vi "CAN read.vi"(8 "error in":errorcluster, 11 "CANopen in":refnum<class "CANopen.lvclass">) -> (0 "error out":errorcluster, 1 "Data":u8[](array[numeric]), 2 "COB-ID":u32, 3 "CANopen out":refnum<class "CANopen.lvclass">, 5 "Time Stamp":timestamp)   [LabVIEW 2024, in "canopen.lvlib" / "CANopen.lvclass"]
doc: "Returns the oldest COB present in the reception queue."
uses:
  CANopen.lvclass
  CANopen.lvclass/CANopen.ctl
  HAL/HAL/Protocols/ICAN/ICAN.lvclass
  HAL/HAL/Time Stamp/Time Stamp.lvclass
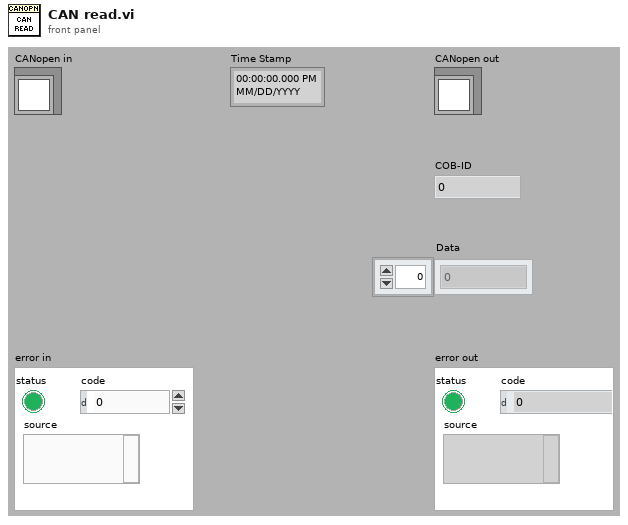
[diagram p1: front panel]
types:
  T1 = cluster{"ID":u32, "MSG type":u8, "DLC":u8, "Time Stamp":refnum<class "Time Stamp.lvclass">, "DATA":u8[]}
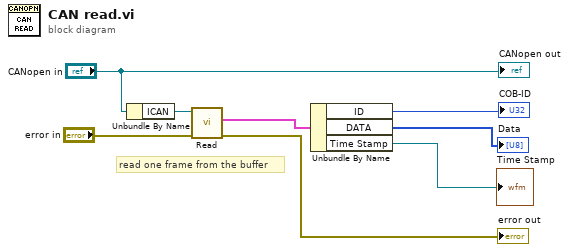
[diagram p0: block diagram]
diagram:
  # "read one frame from the buffer"
  n1 = Unbundle By Name("CANopen in") -> ("ICAN"=w8:refnum<class "ICAN.lvclass">)
  n2 = call-dynamic "Read.vi"("error in"="error in", "ICAN in"=w8) -> ("error out"=→"error out":errorcluster, "CAN Message"=w7:T1)  [unwired: 7 in, 1 out]
  n3 = Unbundle By Name(w7) -> ("ID"=→"COB-ID":u32, "DATA"=→"Data":u8[], "Time Stamp"=→"Time Stamp":refnum<class "Time Stamp.lvclass">)
  "CANopen out" <- "CANopen in"
